vi "ge_GetAllMems.vi"(7 "Rate Class":T1, 10 "Chassis Name":tag, 11 "Config Grandmaster":T2) -> (2 "Taken Dual Rate Mods":string[](array[string]), 3 "All Members":string[](array[string]))   [LabVIEW 2011]
uses:
  Custom Ctrls/Master Cfg/ge_CfgGrandmaster.ctl
  Custom Ctrls/ge_ChassisType.ctl
  Custom Ctrls/Master Cfg/ge_AllGrpTiming.ctl
  Custom Ctrls/ge_LockToLS.ctl
  Custom Ctrls/Master Cfg/ge_GrpTimingCfg.ctl
  Custom Ctrls/Master Cfg/ge_ModBusURLs.ctl
  Custom Ctrls/Master Cfg/ge_ChannelGroup.ctl
  Custom Ctrls/ge_MeasType.ctl
  Classes/Channel/Channel.lvclass
  Custom Ctrls/ge_TimingEngine.ctl
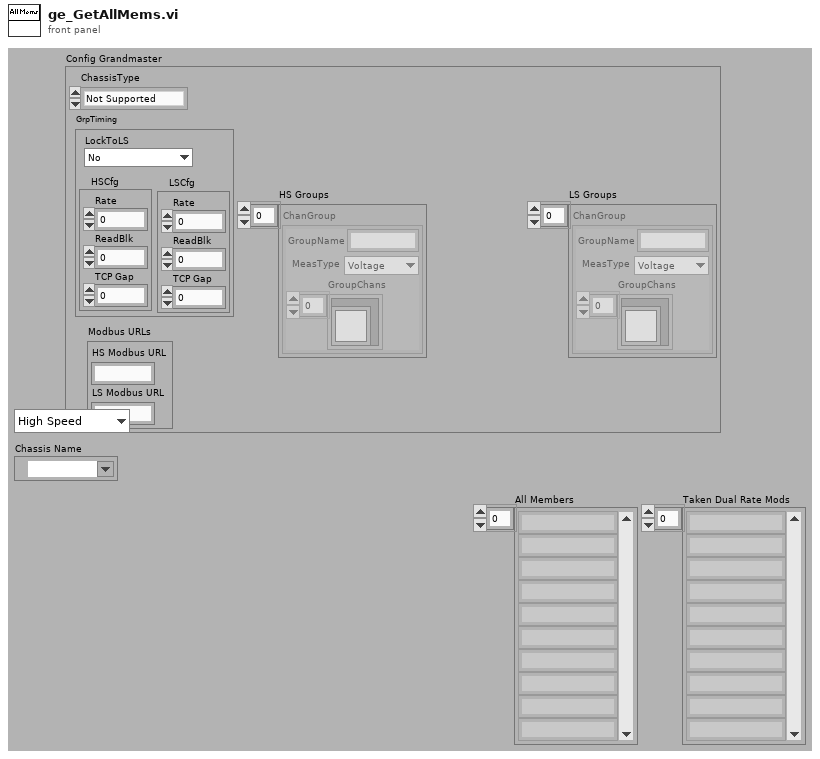
[diagram p1: front panel]
types:
  T1 = typedef "ge_TimingEngine.ctl" = enum16{"High Speed", "Low Speed"}
  T2 = typedef "ge_CfgGrandmaster.ctl" = cluster{"ChassisType":T3, "GrpTiming":T4, "Modbus URLs":T7, "HS Groups":T8[], "LS Groups":T8[]}
  T3 = typedef "ge_ChassisType.ctl" = enum16{"Not Supported", "1-Slot", "4-Slot", "8-Slot"}
  T4 = typedef "ge_AllGrpTiming.ctl" = cluster{"LockToLS":T5, "HSCfg":T6, "LSCfg":T6}
  T5 = typedef "ge_LockToLS.ctl" = enum16{"No", "250ms", "500ms", "1s"}
  T6 = typedef "ge_GrpTimingCfg.ctl" = cluster{"Rate":dbl, "ReadBlk":i32, "TCP Gap":i32}
  T7 = typedef "ge_ModBusURLs.ctl" = cluster{"HS Modbus URL":string, "LS Modbus URL":string}
  T8 = typedef "ge_ChannelGroup.ctl" = cluster{"GroupName":string, "MeasType":T9, "GroupChans":refnum<class "Channel.lvclass">[]}
  T9 = typedef "ge_MeasType.ctl" = enum16{"Voltage", "Frequency", "Tachometer", "Dynamic", "Thermocouple", "RTD", "Strain", "Current", "Resistance"}
  T10 = typedef "ge_MultiRateMods.ctl" = cluster{"NI 9205":bool, "NI 9221":bool}
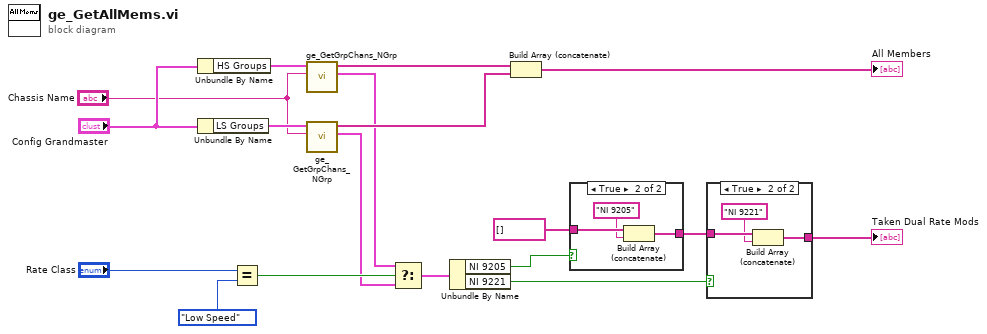
[diagram p0: block diagram]
diagram:
  n1 = Unbundle By Name("Config Grandmaster") -> ("HS Groups"=w18:T8[])
  n2 = Unbundle By Name("Config Grandmaster") -> ("LS Groups"=w12:T8[])
  n3 = Equal?(x="Rate Class", y=ge_TimingEngine."Low Speed") -> (x = y?=w8:bool)
  n4 = call "ge_GetGrpChans_NGrp.vi"("Chassis Name"="Chassis Name", "HS Groups"=w18) -> ("Multi Rate Mods in Grp"=w7:T10, "All Rate Chans"=w16:string[])  [unwired: 7 in, 1 out]
  n5 = call "ge_GetGrpChans_NGrp.vi"("Chassis Name"="Chassis Name", "HS Groups"=w12) -> ("Multi Rate Mods in Grp"=w6:T10, "All Rate Chans"=w11:string[])  [unwired: 7 in, 1 out]
  n6 = Select(t=w7, s=w8, f=w6) -> (s? t:f=w5:T10)
  n7 = Unbundle By Name(w5) -> ("NI 9205"=w4:bool, "NI 9221"=w3:bool)
  n8 = Build Array (concatenate)(w16, w11) -> (→"All Members":string[])
  n9 = case shown="True" w4 {
    tunnel: string[] [] -> [w19 w22]
    tunnel: [w19 w20] -> w13
    frame False {
    }
    frame True {
      n10 = Build Array (concatenate)(w22, "NI 9205") -> (w20:string[])
    }
  }
  n11 = case shown="True" w3 {
    tunnel: w13 -> [w23 w26]
    tunnel: [w23 w24] -> w2
    frame False {
    }
    frame True {
      n12 = Build Array (concatenate)(w26, "NI 9221") -> (w24:string[])
    }
  }
  "Taken Dual Rate Mods" <- w2
